vi "Analyze.vi"(7 "ROI":T1 {"Contours"."Type" items=["No Selection", "Point", "Line", "Rectangle", "Oval", "Polygon", "Freehand Region", "Annulus", "Unused2", "Unused3", "Broken Line", "Freehand Line", "Rotated Rectangle"]}, 8 "error in":errorcluster, 10 "Image in":T2, 11 "State in":T3 caption="State" {"ROI"."Contours"."Type" items=["No Selection", "Point", "Line", "Rectangle", "Oval", "Polygon", "Freehand Region", "Annulus", "Unused2", "Unused3", "Broken Line", "Freehand Line", "Rotated Rectangle"]}) -> (0 "error out":errorcluster, 2 "Image out":T2, 3 "State out":T3 caption="State" {"ROI"."Contours"."Type" items=["No Selection", "Point", "Line", "Rectangle", "Oval", "Polygon", "Freehand Region", "Annulus", "Unused2", "Unused3", "Broken Line", "Freehand Line", "Rotated Rectangle"]})   [LabVIEW 2009, in "POLARIS IMAQ Display.xctl"]
uses:
  POLARIS IMAQ Display.xctl
  State.ctl
  IMAQdx Cam/IMAQdx Cam.lvclass
  Properties/ImageSource.ctl
  <vilib>/vision/Image Controls.llb/IMAQ Image.ctl
  DisplaySettings.ctl
  Named ROI.ctl
  Analyze Classes/Analyze BaseClass/Analyze BaseClass.lvclass
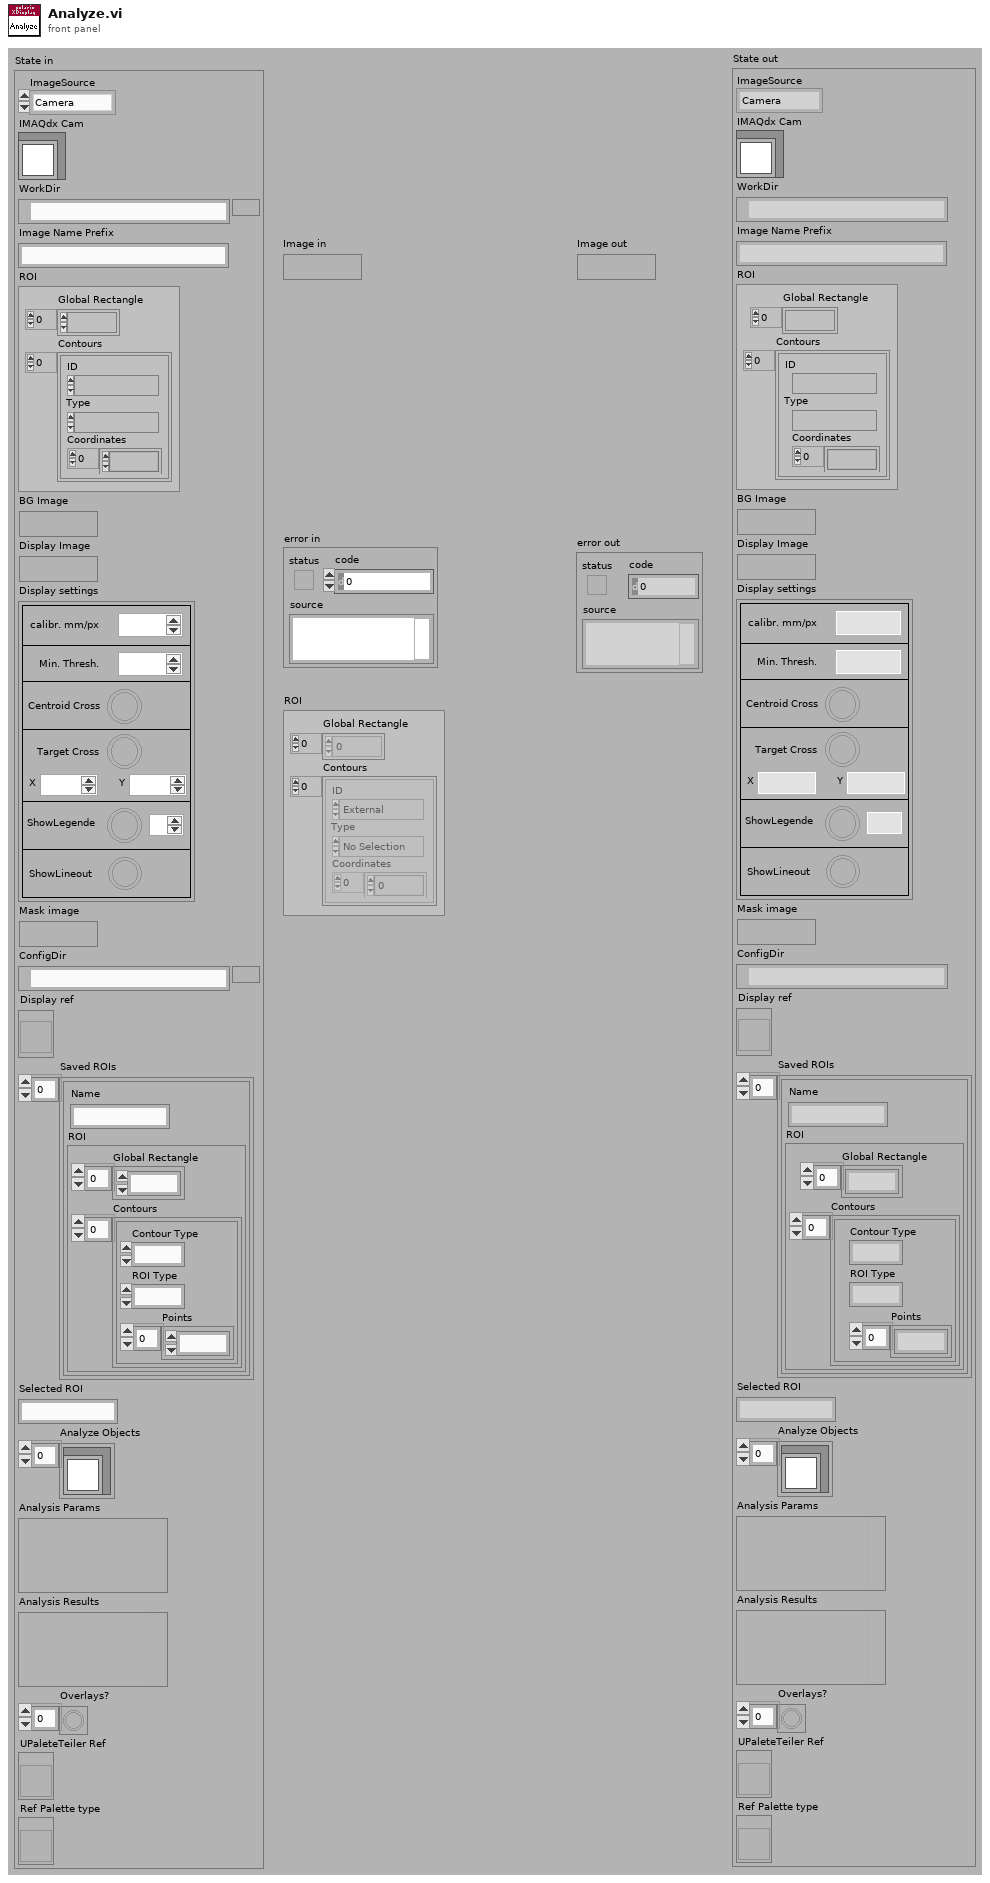
[diagram p1: front panel]
types:
  T1 = typedef "ROI Descriptor" = cluster{"Global Rectangle":i32[], "Contours":cluster{"ID":enum32{"External", "Internal"}, "Type":u32, "Coordinates":i32[]}[]}
  T2 = typedef "IMAQ Image.ctl" = refnum<image>
  T3 = typedef "POLARIS IMAQ Display.xctl/State.ctl" = cluster{"ImageSource":T4, "IMAQdx Cam":refnum<class "IMAQdx Cam.lvclass">, "WorkDir":path, "Image Name Prefix":string, "ROI":T1, "BG Image":T2, "Display Image":T2, "Display settings":T5, "Mask image":T2, "ConfigDir":path, "Display ref":refnum<vi>, "Saved ROIs":T6[], "Selected ROI":string, "Analyze Objects":refnum<class "Analyze BaseClass.lvclass">[], "Analysis Params":variant, "Analysis Results":variant, "Overlays?":bool[], "UPaleteTeiler Ref":refnum<vi>, "Ref Palette type":refnum<vi>}
  T4 = typedef "POLARIS IMAQ Display.xctl/ImageSource.ctl" = enum16{"Camera", "File"}
  T5 = typedef "POLARIS IMAQ Display.xctl/DisplaySettings.ctl" = cluster{"Min. Thresh.":sgl, "X":dbl, "Y":dbl, "ShowLineout":bool, "ScaleParts":i32, "ShowLegende":bool, "Target Cross":bool, "Centroid Cross":bool, "Target color":u32, "Centroid color":u32, "calibr. mm/px":sgl}
  T6 = typedef "POLARIS IMAQ Display.xctl/Named ROI.ctl" = cluster{"ROI":cluster{"Global Rectangle":i32[], "Contours":cluster{"Contour Type":u32, "ROI Type":u32, "Points":i32[]}[]}, "Name":string}
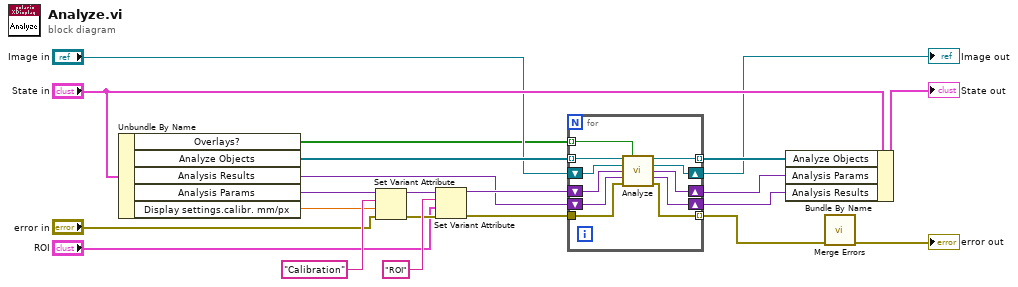
[diagram p0: block diagram]
diagram:
  n1 = Unbundle By Name("State in") -> ("Overlays?"=w1:bool[], "Analyze Objects"=w22:refnum<class "Analyze BaseClass.lvclass">[], "Analysis Results"=w2:variant, "Analysis Params"=w4:variant, "Display settings.calibr. mm/px"=w3:sgl)
  n2 = Set Variant Attribute(Variant=w4, name="Calibration", value=w3, error in="error in") -> (Variant out=w17:variant, error out=w16:errorcluster)  [unwired: 1 out]
  n3 = Set Variant Attribute(Variant=w17, name="ROI", value="ROI", error in=w16) -> (Variant out=w12:variant, error out=w11:errorcluster)  [unwired: 1 out]
  n4 = for {
    tunnel: w22 -> [w33] mode=indexing
    shift-right: [w31] -> w9
    shift-left: "Image in" -> [w28]
    shift-right: [w26] -> w6
    shift-left: w12 -> [w27]
    tunnel: w11 -> [w30]
    tunnel: [w32] -> w10 mode=indexing
    tunnel: [w29] -> w8 mode=indexing
    shift-right: [w24] -> w5
    shift-left: w2 -> [w25]
    tunnel: w1 -> [w23] mode=indexing
    n5 = call-dynamic "Analyze.vi"("Analyze BaseClass in"=w33, "Create Overlay?"=w23, "Image in"=w28, "Parameters"=w27, "Results in"=w25, "error in (no error)"=w30) -> ("Analyze BaseClass out"=w32:refnum<class "Analyze BaseClass.lvclass">, "Image out"=w31:T2, "Parameters out"=w26:variant, "Results"=w24:variant, "error out"=w29:errorcluster)  [unwired: 5 in]
  }
  "Image out" <- w9
  n6 = Bundle By Name(cluster="State in", "Analyze Objects"=w10, "Analysis Params"=w6, "Analysis Results"=w5) -> (→"State out":T3)
  n7 = call <vilib>:"Merge Errors.vi"("error array in"=w8) -> ("error out"=→"error out":errorcluster)  [unwired: 6 in]
